vi "Controle_da_mesa_v2.vi"() -> ()   [LabVIEW 2017]
uses:
  <vilib>/Platform/TimedLoop/XDataNode/timing_clust.ctl
  <vilib>/Platform/TimedLoop/XDataNode/nitl_modes.ctl
  <vilib>/Platform/TimedLoop/XDataNode/wakeup.ctl
  <vilib>/Analysis/_algsub.llb/Real PseudoInverse Matrix.vi
  <vilib>/Analysis/baseanly.llb/Real A x B.vi
  <vilib>/Analysis/Matrix/Numeric/Conversions/Array To Matrix - RA2.vi
  <vilib>/Analysis/Matrix/Numeric/Conversions/Array To Matrix - RA.vi
  <vilib>/Analysis/Matrix/Numeric/Conversions/Matrix To Array - RM.vi
  <vilib>/Platform/TimedLoop/XDataNode/XDataNode.xnode
  <vilib>/Platform/TimedLoop/XDataNode/XDNodeRunTimeDep.lvlib
  <vilib>/Analysis/Matrix/NI_Matrix.lvlib
  <vilib>/Analysis/NI_AALPro.lvlib
  <vilib>/Analysis/NI_AALBase.lvlib
panel:
  out "outer previsto":dbl
  out "inner previsto":dbl
  in  "passo de predição":dbl=0.03 format="%#_13g"
  out "middle previsto":dbl
  out "Period":i64
  out "XY Graph":cluster{dbl[], dbl[]}[](graph)
  in  "Inicia seno":bool
  in  "Inner ON":bool
  in  "Middle ON":bool
  in  "Outer ON":bool
  in  "Amplitude Inner [deg]":dbl=1.0 format="%#_13g"
  in  "Amplitude Middle [deg]":dbl=1.0 format="%#_13g"
  in  "Amplitude Outer [deg]":dbl=1.0 format="%#_13g"
  in  "f inner [Hz]":dbl=1.0 format="%#_13g"
  in  "f middle [Hz]":dbl=1.0 format="%#_13g"
  in  "f outer [Hz]":dbl=1.0 format="%#_13g"
  out "spreadsheet string":string
  in  "UTC format":bool
  out "appended path":path
  out "concatenated string":string
  out "ACCEL":cluster{dbl, dbl, dbl} {"?" format="%1_6g"}
  out "RATE":cluster{dbl, dbl, dbl} {"?" format="%1_6g"}
  out "POS":cluster{dbl, dbl, dbl} {"?" format="%_6g"; "?" format="%#1_6g"}
  out "Tempo (s)":dbl
  out "string enviada para acutrol":string
  in  "Remote Host":string="192.168.53.1"
  in  "Para Controle da mesa":bool
  # "Atentar-se para que a posição inicial da mesa seja a mesma posição comandada. (Condições iniciais - Pos/Rate/Accel)"
  # "Monitor"
  # "Inner"
  # "Middle"
  # "Outer"
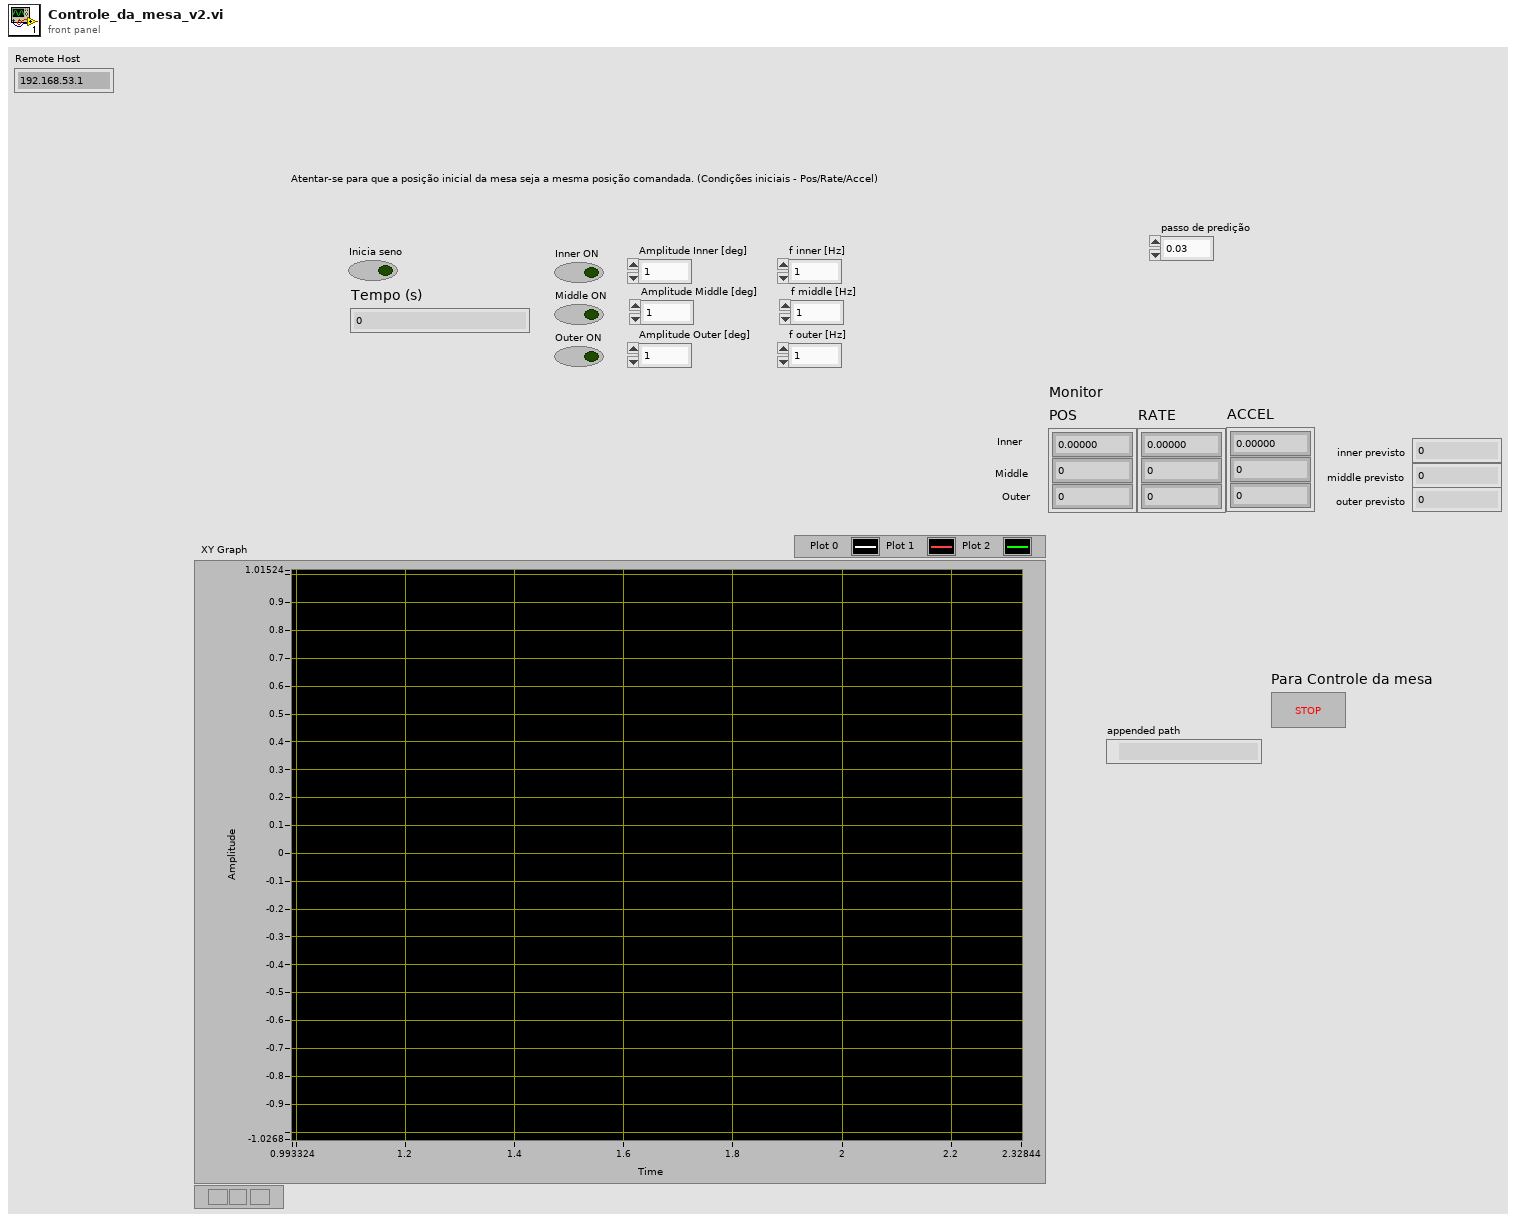
[diagram p1: front panel]
types:
  T1 = enum16{"open", "replace", "create", "open or create", "replace or create", "replace or create with confirmation"}
  T2 = typedef "XDNodeRunTimeDep.lvlib/timing_clust.ctl" = cluster{"Expected End [f-1]":u64, "Actual End [f-1]":u64, "Finished Late? [f-1]":bool, "Expected End [i-1]":u64, "Actual End [i-1]":u64, "Finished Late? [i-1]":bool, "Expected Start [i]":u64, "Actual Start [i]":u64, "Expected Start [f]":u64, "Actual Start [f]":u64, "Source Name":string, "Structure Name":string, "Period":i64, "Deadline":i64, "Offset":i64, "Start":i64, "Priority":i32, "Timeout":i32, "Mode":T3, "Wakeup Reason":T4, "Error":errorcluster, "Source Type":string, "Secondary Source Type":string, "Global End Time":u64, "Global Start Time":u64, "Frame Duration":u64, "Iteration Duration":u64, "Assigned CPU":i32, "I/O Scan Engine Mode":u32}
  T3 = typedef "XDNodeRunTimeDep.lvlib/nitl_modes.ctl" = enum32{"No Change", "Process missed periods, maintain original phase", "Discard missed periods, maintain original phase", "Process missed periods, ignore original phase", "Discard missed periods, ignore original phase"}
  T4 = typedef "XDNodeRunTimeDep.lvlib/wakeup.ctl" = enum32{"Normal", "Aborted", "Asynchronous wakeup", "Timing source error", "Timed loop error", "Timeout"}
  T5 = typedef "NI_Matrix.lvlib/RealMatrix.ctl" = dbl[][]
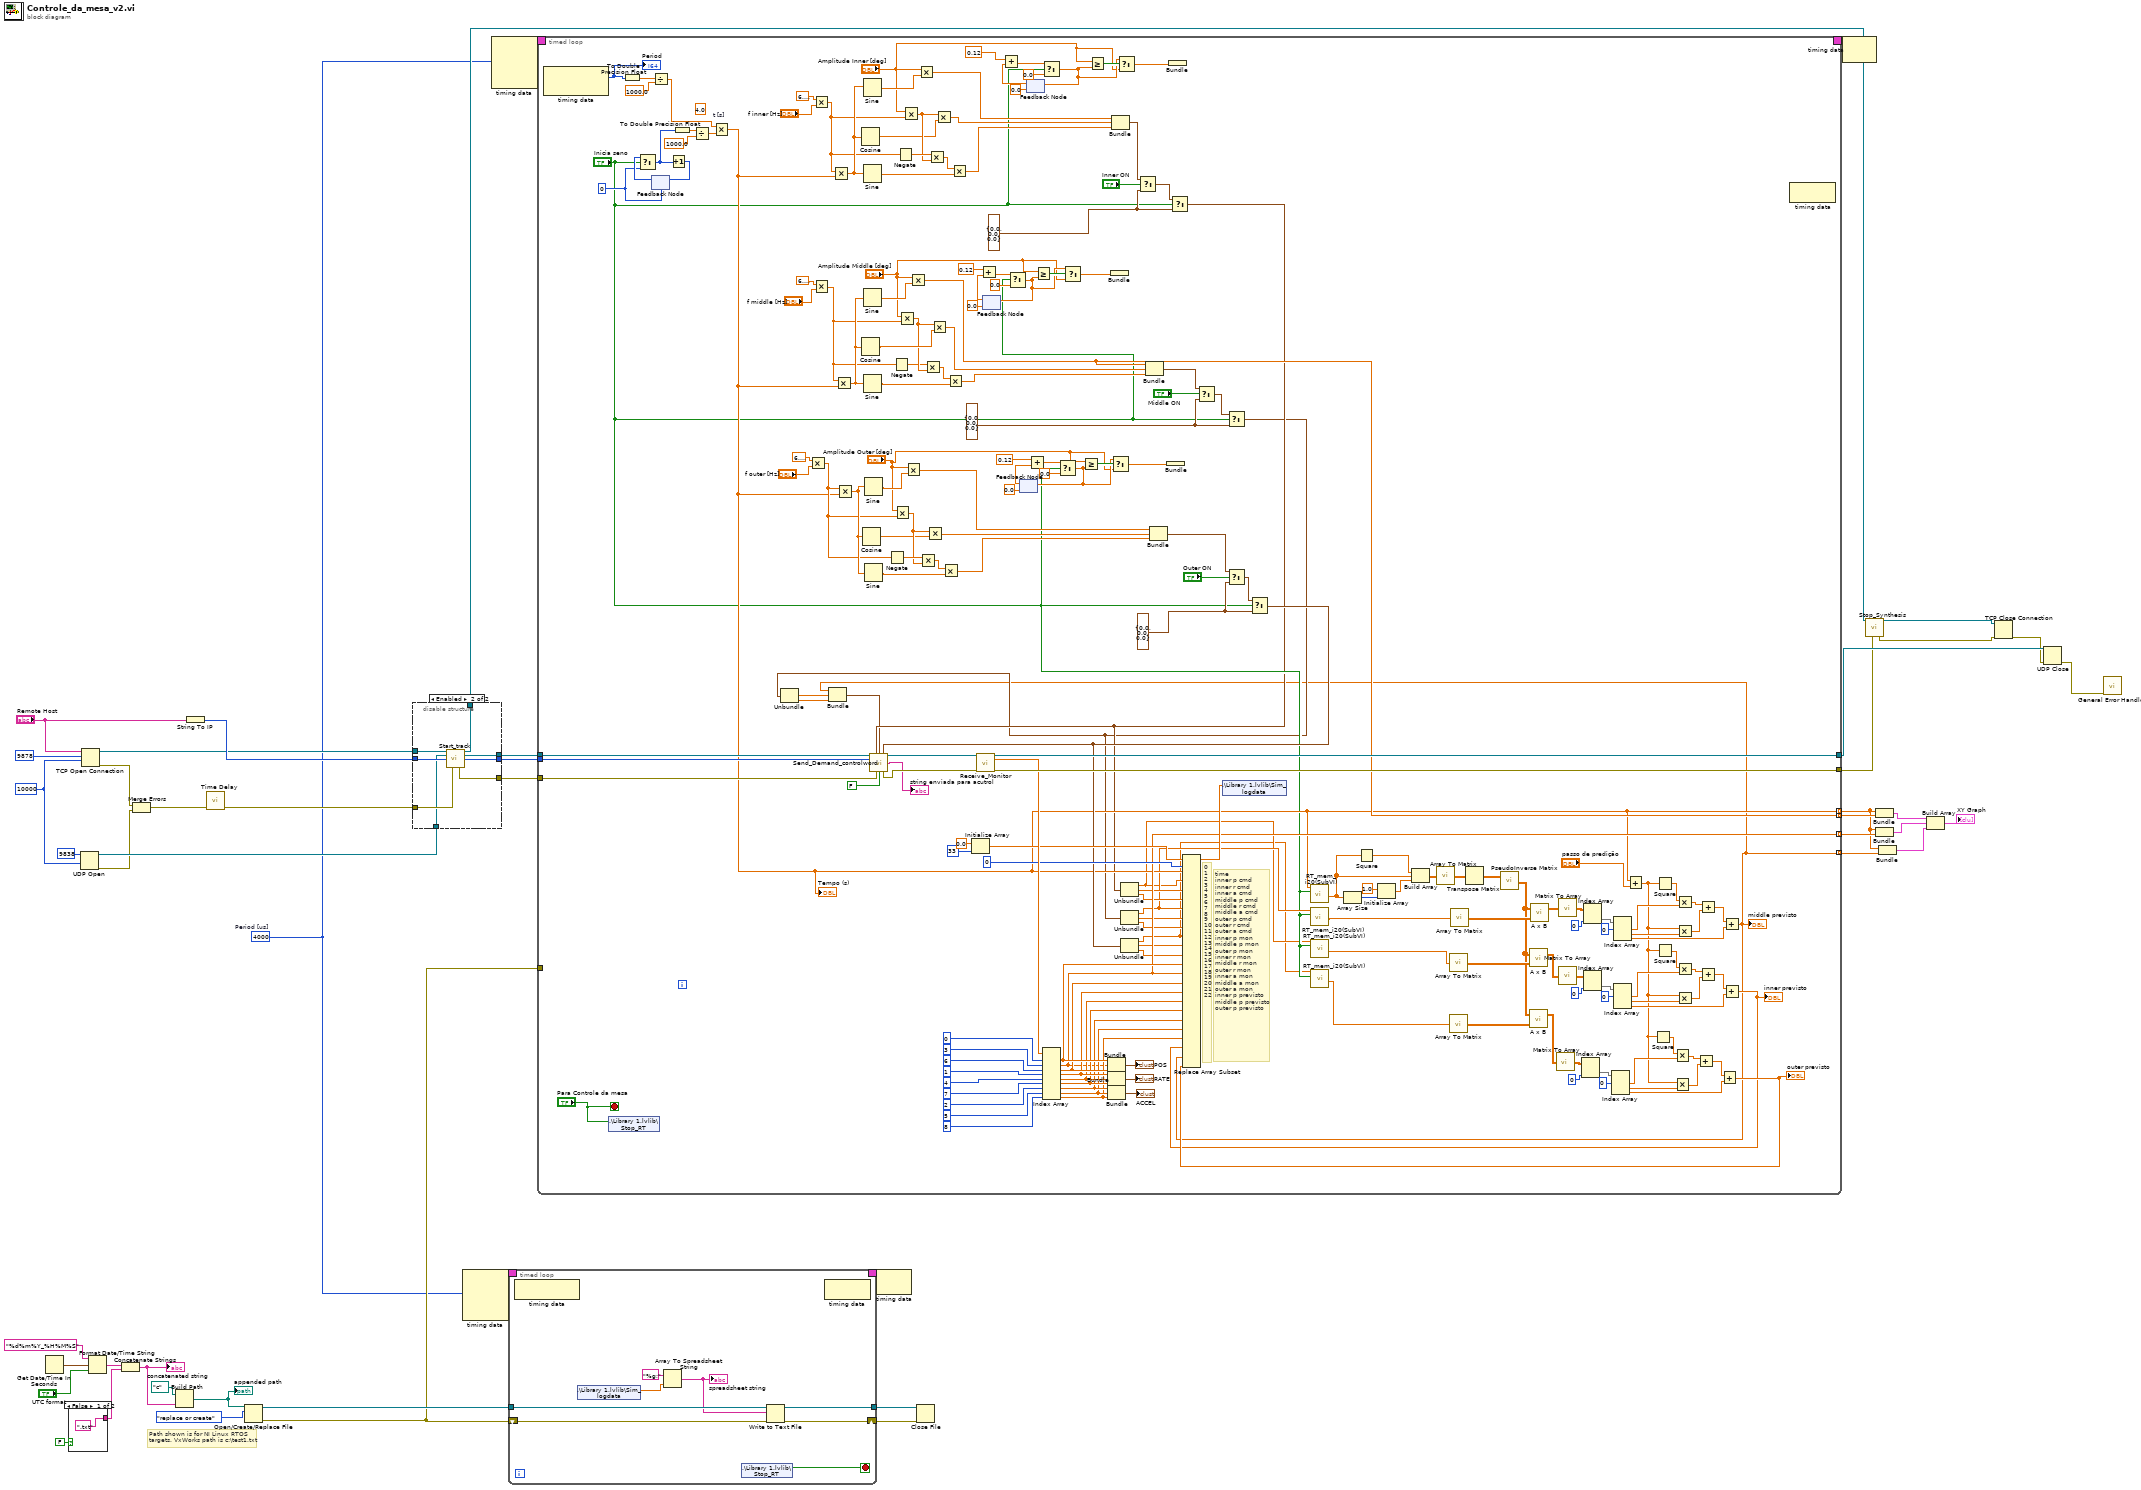
[diagram p0: block diagram]
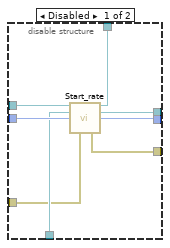
[diagram p2: hidden frame]
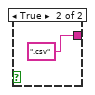
[diagram p3: hidden frame]
diagram:
  w6 = 10000 ("timeout ms (60000)")
  w20 = i64 4000  # Period [us]
  # "Path shown is for NI Linux RTOS\ntargets. VxWorks path is c:\\test1.txt"
  n1 = Get Date/Time In Seconds() -> (seconds since 1Jan1904=w32:timestamp)
  n2 = case shown="False" FALSE {
    tunnel: [".txt" ("string") ".csv" ("string")] -> w36
    frame False {
    }
    frame True {
    }
  }
  n3 = UDP Open(9:w6, 11:u16 9838 ("port")) -> (port=w47:refnum<k16>, 0:w5:errorcluster)  [unwired: 1 in, 3 out]
  n4 = TCP Open Connection(address="Remote Host", remote port or service name=u16 9878, timeout ms (60000)=w6) -> (connection ID=w46:refnum<k5>, error out=w7:errorcluster)  [unwired: 2 in]
  n5 = Format Date/Time String(time format string (%c)="%d%m%Y_%H%M%S", seconds (now)=w32, UTC format="UTC format") -> (date/time string=w31:string)
  n6 = Concatenate Strings(w31, w36) -> (w37:string)
  "concatenated string" <- w37
  n7 = Merge Errors(w7, w5) -> (w10:errorcluster)
  n8 = Build Path(base path=path "c:/" ("file path (use dialog)"), name or relative path=w37) -> (appended path=w35:path)
  "appended path" <- w35
  n9 = String To IP(1:"Remote Host") -> (0:w48:u32)
  n10 = call "Time Delay"("error in (no error)"=w10) -> ("error out"=w45:errorcluster)  [unwired: 10 in]
  n11 = Open/Create/Replace File(file path (use dialog)=w35, operation (0:open)=T1."replace or create") -> (refnum out=w40:refnum<file>, error out=w21:errorcluster)  [unwired: 4 in, 1 out]
  n12 = disable-structure shown="Enabled" {
    disable-tunnel: w48 -> [w58 w65]
    disable-tunnel: w47 -> [w57 w63]
    disable-tunnel: w46 -> [w56 w66]
    disable-tunnel: w45 -> [w55 w64]
    disable-tunnel: [w54 w61] -> w26
    disable-tunnel: [w53 w60] -> w25
    disable-tunnel: [w52 w59] -> w24
    disable-tunnel: [w51 w62] -> w22
    frame Disabled {
      n13 = call "Start_rate.vi"("TCP connection ID"=w56, "UDP connection ID"=w57, "IP address in"=w58, "error in"=w55) -> ("TCP connection ID out"=w51:refnum<k5>, "UDP connection ID out"=w54:refnum<k16>, "IP address out"=w53:u32, "error out"=w52:errorcluster)  [unwired: 7 in, 1 out]
    }
    frame Enabled {
      n14 = call "Start_track.vi"("TCP connection ID"=w66, "UDP connection ID"=w63, "IP address in"=w65, "error in"=w64) -> ("TCP connection ID out"=w62:refnum<k5>, "UDP connection ID out"=w61:refnum<k16>, "IP address out"=w60:u32, "error out"=w59:errorcluster)  [unwired: 7 in, 1 out]
    }
  }
  n15 = node-c288(w20) -> (w43:T2)  [unwired: 3 in]
  n16 = node-c288(w20) -> (w28:T2)  [unwired: 3 in]
  n17 = timed-loop {
    tunnel: w40 -> [w74]
    tunnel: [w73] -> w39
    timing: w43 -> [_]
    timing-out: [_] -> w42
    shift-right: [w67] -> w30
    shift-left: w21 -> [w68]
    stop <- w72 stop-if-true
    n18 = node-c288() -> ()  [unwired: 1 in, 1 out]
    n19 = shared-variable ".\\Library 1.lvlib\\Sim_logdata"() -> (w70:dbl[])  [unwired: 1 in, 1 out]
    n20 = Array To Spreadsheet String(array=w70, 3:"%g;" ("format string")) -> (spreadsheet string=w69:string)  [unwired: 1 in]
    "spreadsheet string" <- w69
    n21 = shared-variable ".\\Library 1.lvlib\\Stop_RT"() -> (w72:bool)  [unwired: 1 in, 1 out]
    n22 = Write to Text File(file (use dialog)=w74, text=w69, error in=w68) -> (refnum out=w73:refnum<file>, error out=w67:errorcluster)  [unwired: 1 in, 1 out]
    n23 = node-c288() -> ()  [unwired: 1 in, 1 out]
  }
  n24 = timed-loop {
    timing: w28 -> [_]
    timing-out: [_] -> w27
    tunnel: w26 -> [w273]
    tunnel: w25 -> [w272]
    tunnel: w24 -> [w271]
    tunnel: [w275] -> w23
    tunnel: [w274] -> w44
    tunnel: w21 -> [_]
    tunnel: [w131] -> w14 mode=indexing
    tunnel: [w148] -> w19 mode=indexing
    tunnel: [w166] -> w16 mode=indexing
    tunnel: [w77] -> w13 mode=indexing
    stop <- "Para Controle da mesa" stop-if-true
    w201 = cluster{dbl, dbl, dbl} {0.0, 0.0, 0.0} ("f")
    w205 = cluster{dbl, dbl, dbl} {0.0, 0.0, 0.0} ("f")
    w208 = cluster{dbl, dbl, dbl} {0.0, 0.0, 0.0} ("f")
    (unwired) 4.0 ("x")
    w250 = 0
    # "time\ninner p cmd\ninner r cmd\ninner a cmd\nmiddle p cmd\nmiddle r cmd\nmiddle a cmd\nouter p cmd\nouter r cmd\nouter a cmd\ninner p mon\nmiddle p mon\nouter p mon\ninner r mon\nmiddle r mon\nouter r mon\ninner a mon\nmiddle a mon\nouter a mon\ninner p previsto\nmiddle p previsto\nouter p previsto"
    # "0\n1\n2\n3\n4\n5\n6\n7\n8\n9\n10\n11\n12\n13\n14\n15\n16\n17\n18\n19\n20\n21\n22"
    n25 = node-c288() -> (w154:i64)  [unwired: 1 in, 1 out]
    "Period" <- w154
    n26 = shared-variable ".\\Library 1.lvlib\\Stop_RT"("Para Controle da mesa") -> ()  [unwired: 1 in, 1 out]
    n27 = To Double Precision Float(number=w154) -> (double precision float=w155:dbl)
    n28 = feedback #1(w250) -> (w251:i32)
    n29 = Select(t=w251, s="Inicia seno", f=w250) -> (s? t:f=w244:i32)
    n30 = Divide(x=w155, y=1000.0) -> (x/y=w153:dbl)
    n31 = Increment(x=w244) -> (x+1=w249:i32)
    n32 = feedback-in #1(w249) -> ()
    n33 = To Double Precision Float(number=w244) -> (double precision float=w245:dbl)
    n34 = Divide(x=w245, y=1000.0) -> (x/y=w243:dbl)
    n35 = Multiply "t [s]"(x=w153, y=w243) -> (x*y=w131:dbl)
    "Tempo (s)" <- w131
    n36 = Multiply(x=6.283185307179586, y="f outer [Hz]") -> (x*y=w211:dbl)
    n37 = Multiply(x=6.283185307179586, y="f inner [Hz]") -> (x*y=w235:dbl)
    n38 = Multiply(x=6.283185307179586, y="f middle [Hz]") -> (x*y=w212:dbl)
    n39 = Multiply(x=w235, y=w131) -> (x*y=w242:dbl)
    n40 = Multiply(x=w212, y=w131) -> (x*y=w216:dbl)
    n41 = Multiply(x=w211, y=w131) -> (x*y=w213:dbl)
    n42 = Cosine(x=w242) -> (cos(x)=w234:dbl)
    n43 = Cosine(x=w216) -> (cos(x)=w231:dbl)
    n44 = Cosine(x=w213) -> (cos(x)=w220:dbl)
    n45 = Sine(x=w242) -> (sin(x)=w236:dbl)
    n46 = Sine(x=w242) -> (sin(x)=w233:dbl)
    n47 = Sine(x=w216) -> (sin(x)=w230:dbl)
    n48 = Sine(x=w216) -> (sin(x)=w232:dbl)
    n49 = Sine(x=w213) -> (sin(x)=w221:dbl)
    n50 = Sine(x=w213) -> (sin(x)=w219:dbl)
    n51 = Negate(x=w211) -> (-x=w224:dbl)
    n52 = Negate(x=w212) -> (-x=w225:dbl)
    n53 = Multiply(x="Amplitude Outer [deg]", y=w211) -> (x*y=w223:dbl)
    n54 = Negate(x=w235) -> (-x=w241:dbl)
    n55 = Multiply(x="Amplitude Middle [deg]", y=w212) -> (x*y=w226:dbl)
    n56 = Multiply(x="Amplitude Inner [deg]", y=w235) -> (x*y=w240:dbl)
    n57 = Multiply(x="Amplitude Outer [deg]", y=w221) -> (x*y=w147:dbl)
    n58 = Multiply(x="Amplitude Middle [deg]", y=w230) -> (x*y=w148:dbl)
    n59 = Multiply(x="Amplitude Inner [deg]", y=w236) -> (x*y=w149:dbl)
    n60 = Multiply(x=w224, y=w223) -> (x*y=w222:dbl)
    n61 = Multiply(x=w225, y=w226) -> (x*y=w227:dbl)
    n62 = Multiply(x=w223, y=w220) -> (x*y=w164:dbl)
    n63 = Multiply(x=w241, y=w240) -> (x*y=w239:dbl)
    n64 = Multiply(x=w226, y=w231) -> (x*y=w228:dbl)
    n65 = Multiply(x=w240, y=w234) -> (x*y=w238:dbl)
    n66 = Multiply(x=w222, y=w219) -> (x*y=w163:dbl)
    n67 = Multiply(x=w227, y=w232) -> (x*y=w229:dbl)
    n68 = Multiply(x=w239, y=w233) -> (x*y=w237:dbl)
    n69 = Initialize Array(0.0 ("element"), 33 ("dimension size")) -> (w254:dbl[])
    n70 = feedback #2(0.0) -> (w177:dbl)
    n71 = Add(x=0.12, y=w177) -> (x+y=w178:dbl)
    n72 = Select(t=w178, s="Inicia seno", f=0.0) -> (s? t:f=w170:dbl)
    n73 = feedback-in #2(w170) -> ()
    n74 = feedback #3(0.0) -> (w175:dbl)
    n75 = feedback #4(0.0) -> (w173:dbl)
    n76 = Add(x=0.12, y=w173) -> (x+y=w174:dbl)
    n77 = Add(x=0.12, y=w175) -> (x+y=w176:dbl)
    n78 = Greater Or Equal?(x="Amplitude Middle [deg]", y=w170) -> (x >= y?=w187:bool)
    n79 = Select(t=w174, s="Inicia seno", f=0.0) -> (s? t:f=w172:dbl)
    n80 = feedback-in #4(w172) -> ()
    n81 = Select(t=w176, s="Inicia seno", f=0.0) -> (s? t:f=w168:dbl)
    n82 = feedback-in #3(w168) -> ()
    n83 = Select(t=w170, s=w187, f="Amplitude Middle [deg]") -> (s? t:f=w151:dbl)
    n84 = Greater Or Equal?(x="Amplitude Outer [deg]", y=w168) -> (x >= y?=w182:bool)
    n85 = Greater Or Equal?(x="Amplitude Inner [deg]", y=w172) -> (x >= y?=w188:bool)
    n86 = Bundle("Amplitude Middle [deg]"=w151) -> ()  [unwired: 1 in, 1 out]
    n87 = Bundle(w149, w238, w237) -> (w209:cluster{dbl, dbl, dbl})  [unwired: 1 in]
    n88 = Select(t=w168, s=w182, f="Amplitude Outer [deg]") -> (s? t:f=w150:dbl)
    n89 = Select(t=w172, s=w188, f="Amplitude Inner [deg]") -> (s? t:f=w152:dbl)
    n90 = Select(t=w209, s="Inner ON", f=w208) -> (s? t:f=w207:cluster{dbl, dbl, dbl})
    n91 = Bundle(w148, w228, w229) -> (w204:cluster{dbl, dbl, dbl})  [unwired: 1 in]
    n92 = Bundle(w147, w164, w163) -> (w200:cluster{dbl, dbl, dbl})  [unwired: 1 in]
    n93 = Bundle("Amplitude Outer [deg]"=w150) -> ()  [unwired: 1 in, 1 out]
    n94 = Bundle("Amplitude Inner [deg]"=w152) -> ()  [unwired: 1 in, 1 out]
    n95 = Select(t=w207, s="Inicia seno", f=w208) -> (s? t:f=w80:cluster{dbl, dbl, dbl})
    n96 = Unbundle(w80) -> (w120:dbl, w162:dbl, w161:dbl)
    n97 = Select(t=w204, s="Middle ON", f=w205) -> (s? t:f=w203:cluster{dbl, dbl, dbl})
    n98 = Select(t=w203, s="Inicia seno", f=w205) -> (s? t:f=w78:cluster{dbl, dbl, dbl})
    n99 = Unbundle(w78) -> (w82:dbl, w81:dbl)  [unwired: 1 out]
    n100 = Unbundle(w78) -> (w122:dbl, w160:dbl, w159:dbl)
    n101 = Select(t=w200, s="Outer ON", f=w201) -> (s? t:f=w199:cluster{dbl, dbl, dbl})
    n102 = Select(t=w199, s="Inicia seno", f=w201) -> (s? t:f=w165:cluster{dbl, dbl, dbl})
    n103 = Unbundle(w165) -> (w119:dbl, w158:dbl, w157:dbl)
    n104 = call "RT_mem_i20(SubVI).vi"("start"="Inicia seno", "In"=w131) -> ("in_vec"=w143:dbl[])  [unwired: 8 in, 1 out]
    n105 = call "RT_mem_i20(SubVI).vi"("start"="Inicia seno", "In"=w122) -> ("in_vec"=w123:dbl[])  [unwired: 8 in, 1 out]
    n106 = call "RT_mem_i20(SubVI).vi"("start"="Inicia seno", "In"=w120) -> ("in_vec"=w116:dbl[])  [unwired: 8 in, 1 out]
    n107 = call "RT_mem_i20(SubVI).vi"("start"="Inicia seno", "In"=w119) -> ("in_vec"=w115:dbl[])  [unwired: 8 in, 1 out]
    n108 = Array Size(array=w143) -> (size(s)=w146:i32)
    n109 = Square(x=w143) -> (x^2=w144:dbl[])
    n110 = Initialize Array(1.0 ("element"), w146) -> (w142:dbl[])
    n111 = Build Array(w144, w143, w142) -> (w140:dbl[][])
    n112 = call-poly <vilib>:"Array To Matrix.vi"("Real 2D Array"=w140) -> ("Real Matrix"=w141:T5)
    n113 = call-poly <vilib>:"Array To Matrix.vi"("Real 1D Array"=w116) -> ("Real Matrix (Column Vector)"=w118:T5)
    n114 = call-poly <vilib>:"Array To Matrix.vi"("Real 1D Array"=w115) -> ("Real Matrix (Column Vector)"=w117:T5)
    n115 = call-poly <vilib>:"Array To Matrix.vi"("Real 1D Array"=w123) -> ("Real Matrix (Column Vector)"=w138:T5)
    n116 = Transpose Matrix(1:w141) -> (0:w139:T5)
    n117 = call-poly <vilib>:"PseudoInverse Matrix.vi"("Input Matrix"=w139) -> ("PseudoInverse Matrix"=w92:T5)  [unwired: 1 in, 1 out]
    n118 = call-poly <vilib>:"A x B.vi"("B"=w118, "A"=w92) -> ("A x B"=w91:T5)  [unwired: 1 out]
    n119 = call-poly <vilib>:"A x B.vi"("B"=w117, "A"=w92) -> ("A x B"=w90:T5)  [unwired: 1 out]
    n120 = call-poly <vilib>:"A x B.vi"("B"=w138, "A"=w92) -> ("A x B"=w135:T5)  [unwired: 1 out]
    n121 = call-poly <vilib>:"Matrix To Array.vi"("Real Matrix"=w90) -> ("Real 2D Array"=w103:dbl[][])
    n122 = call-poly <vilib>:"Matrix To Array.vi"("Real Matrix"=w135) -> ("Real 2D Array"=w137:dbl[][])
    n123 = call-poly <vilib>:"Matrix To Array.vi"("Real Matrix"=w91) -> ("Real 2D Array"=w104:dbl[][])
    n124 = Index Array(array=w103, index (col)=0 ("index (row)")) -> (element=w101:dbl[])  [unwired: 1 in]
    n125 = Index Array(array=w137, index (col)=0 ("index (row)")) -> (element=w134:dbl[])  [unwired: 1 in]
    n126 = Index Array(array=w104, index (col)=0 ("index (row)")) -> (element=w106:dbl[])  [unwired: 1 in]
    n127 = Index Array(array=w101, index #1=0 ("index")) -> (element #1=w98:dbl, element #2=w96:dbl, element #3=w93:dbl)  [unwired: 2 in]
    n128 = Index Array(array=w134, index #1=0 ("index")) -> (element #1=w129:dbl, element #2=w127:dbl, element #3=w124:dbl)  [unwired: 2 in]
    n129 = Index Array(array=w106, index #1=0 ("index")) -> (element #1=w109:dbl, element #2=w111:dbl, element #3=w114:dbl)  [unwired: 2 in]
    n130 = Add(x=w131, y="passo de predição") -> (x+y=w89:dbl)
    n131 = Square(x=w89) -> (x^2=w99:dbl)
    n132 = Square(x=w89) -> (x^2=w130:dbl)
    n133 = Square(x=w89) -> (x^2=w108:dbl)
    n134 = Multiply(x=w99, y=w98) -> (x*y=w97:dbl)
    n135 = Multiply(x=w89, y=w96) -> (x*y=w95:dbl)
    n136 = Multiply(x=w130, y=w129) -> (x*y=w128:dbl)
    n137 = Multiply(x=w89, y=w127) -> (x*y=w126:dbl)
    n138 = Multiply(x=w108, y=w109) -> (x*y=w110:dbl)
    n139 = Multiply(x=w89, y=w111) -> (x*y=w112:dbl)
    n140 = Add(x=w97, y=w95) -> (x+y=w94:dbl)
    n141 = Add(x=w128, y=w126) -> (x+y=w125:dbl)
    n142 = Add(x=w110, y=w112) -> (x+y=w113:dbl)
    n143 = Add(x=w94, y=w93) -> (x+y=w84:dbl)
    "outer previsto" <- w84
    n144 = Add(x=w125, y=w124) -> (x+y=w77:dbl)
    "middle previsto" <- w77
    n145 = Bundle(w77, w82, w81) -> (w79:cluster{dbl, dbl, dbl})  [unwired: 1 in]
    n146 = call "Send_Demand_controlword.vi"("UDP connection ID out"=w273, "Inner TRACK"=w80, "Middle TRACK"=w79, "Outer TRACK"=w165, "IP address in"=w272, "error in"=w271, "ReadOnly"=FALSE) -> ("UDP connection ID out"=w86:refnum<k16>, "concatenated string"=→"string enviada para acutrol":string, "error out"=w88:errorcluster)  [unwired: 5 in, 1 out]
    n147 = call "Receive_Monitor.vi"("UDP connection ID"=w86, "error out 2"=w88) -> ("UDP connection ID out"=w274:refnum<k16>, "MonitorBlock"=w262:dbl[], "error out"=w275:errorcluster)  [unwired: 11 in]
    n148 = Index Array(array=w262, index #1=0 ("index"), index #2=3 ("index"), index #3=6 ("index"), index #4=1 ("index"), index #5=4 ("index"), index #6=7 ("index"), index #7=2 ("index"), index #8=5 ("index"), index #9=8 ("index")) -> (element #1=w198:dbl, element #2=w166:dbl, element #3=w197:dbl, element #4=w196:dbl, element #5=w195:dbl, element #6=w194:dbl, element #7=w193:dbl, element #8=w192:dbl, element #9=w191:dbl)
    n149 = Bundle(w198, w166, w197) -> (→"POS":cluster{dbl, dbl, dbl})  [unwired: 1 in]
    n150 = Bundle(w196, w195, w194) -> (→"RATE":cluster{dbl, dbl, dbl})  [unwired: 1 in]
    n151 = Bundle(w193, w192, w191) -> (→"ACCEL":cluster{dbl, dbl, dbl})  [unwired: 1 in]
    n152 = Add(x=w113, y=w114) -> (x+y=w83:dbl)
    "inner previsto" <- w83
    n153 = Replace Array Subset(array=w254, new element #1=w131, index #1=0 ("index"), new element #2=w120, new element #3=w162, new element #4=w161, new element #5=w122, new element #6=w160, new element #7=w159, new element #8=w119, new element #9=w158, new element #10=w157, new element #11=w198, new element #12=w166, new element #13=w197, new element #14=w196, new element #15=w195, new element #16=w194, new element #17=w193, new element #18=w192, new element #19=w191, new element #20=w83, new element #21=w77, new element #22=w84) -> (w253:dbl[])  [unwired: 21 in]
    n154 = shared-variable ".\\Library 1.lvlib\\Sim_logdata"(w253) -> ()  [unwired: 1 in, 1 out]
    n155 = node-c288() -> ()  [unwired: 1 in, 1 out]
  }
  n156 = node-c288(w42) -> ()  [unwired: 1 out]
  n157 = Close File(refnum=w39, error in=w30) -> ()  [unwired: 2 out]
  n158 = node-c288(w27) -> ()  [unwired: 1 out]
  n159 = call "Stop_Synthesis.vi"("TCP connection ID"=w22, "error in"=w23) -> ("TCP connection ID out"=w3:refnum<k5>, "error out"=w2:errorcluster)  [unwired: 12 in]
  n160 = Bundle(w14, w19) -> (w18:cluster{dbl[], dbl[]})  [unwired: 1 in]
  n161 = Bundle(w14, w16) -> (w17:cluster{dbl[], dbl[]})  [unwired: 1 in]
  n162 = Bundle(w14, w13) -> (w12:cluster{dbl[], dbl[]})  [unwired: 1 in]
  n163 = Build Array(w18, w17, w12) -> (→"XY Graph":cluster{dbl[], dbl[]}[])
  n164 = TCP Close Connection(connection ID=w3, error in (no error)=w2) -> (error out=w1:errorcluster)  [unwired: 1 in, 1 out]
  n165 = UDP Close(connection ID=w44, 8:w1) -> (error out=w4:errorcluster)  [unwired: 1 out]
  n166 = call <vilib>:"General Error Handler.vi"("error in (no error)"=w4) -> ()  [unwired: 2 in, 13 out]
